vi "SPI_Read_protocol.vi"(0 "Register_adress":bool[](array[boolean])=[FALSE, FALSE, FALSE, FALSE, FALSE, FALSE, FALSE, FALSE, FALSE, FALSE, FALSE, FALSE, FALSE, FALSE, FALSE, FALSE, FALSE, FALSE, FALSE, FALSE, FALSE, FALSE, FALSE, FALSE, FALSE, FALSE, FALSE, FALSE, FALSE, FALSE, FALSE, FALSE], 1 "bit_index":i32, 3 "rising_edge":bool) -> (7 "SDO_Msg":bool)   [LabVIEW 2019]
doc: "This Vi Read a slave message based on SPI protocol. It works with a clock handler and inside a loop"
uses:
  <vilib>/rvi/eio/common/nirviEmuTemplateMethod_errors.vi
  <vilib>/eio/EIONode/EIONode.xnode
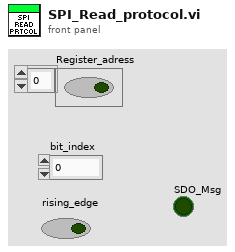
[diagram p1: front panel]
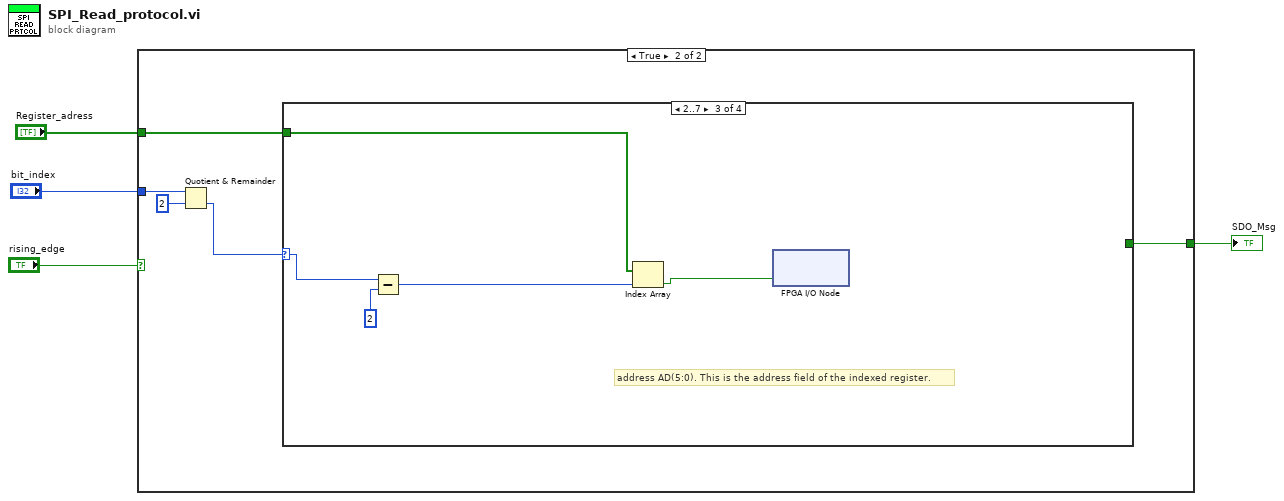
[diagram p0: block diagram]
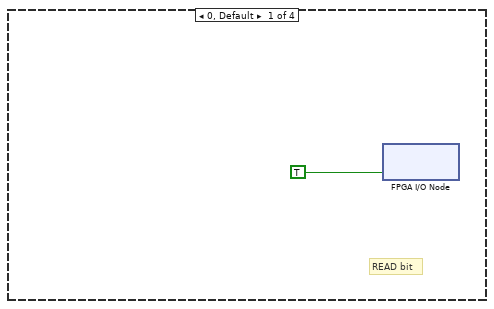
[diagram p3: hidden frame]
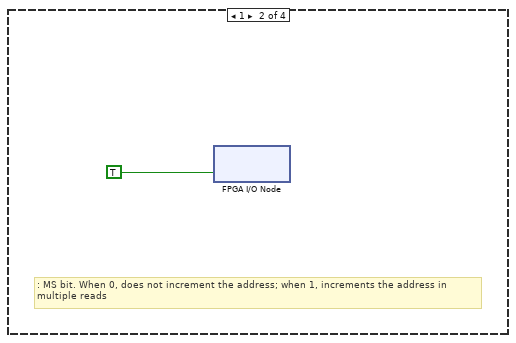
[diagram p4: hidden frame]
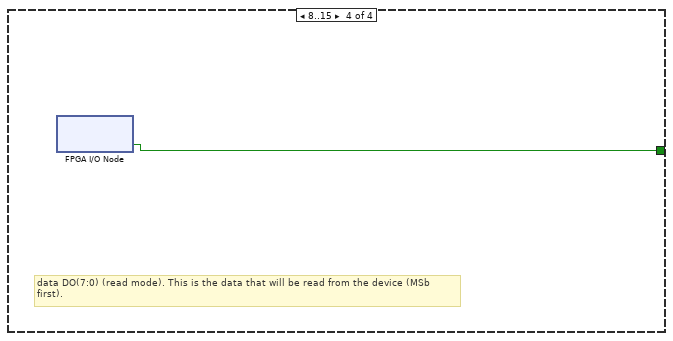
[diagram p5: hidden frame]
diagram:
  n1 = case shown="True" "rising_edge" {
    tunnel: "bit_index" -> [_ w8]
    tunnel: [_ w9] -> w2
    tunnel: "Register_adress" -> [_ w5]
    frame False {
    }
    frame True {
      n2 = Quotient & Remainder(x=w8, y=2) -> (floor(x/y)=w6:i32)  [unwired: 1 out]
      n3 = case shown="2..7" w6 {
        selector: w6 -> [_ _ w16 _]
        tunnel: [_ _ _ w17] -> w9
        tunnel: w5 -> [_ _ w13 _]
        frame 0, Default {
          # "READ bit"
          n4 = xnode "FPGA I/O Node"("SDI"=TRUE) -> ()  [unwired: 1 in, 1 out]
        }
        frame 1 {
          # ": MS bit. When 0, does not increment the address; when 1, increments the address in\nmultiple reads"
          n5 = xnode "FPGA I/O Node"("SDI"=TRUE) -> ()  [unwired: 1 in, 1 out]
        }
        frame 2..7 {
          # "address AD(5:0). This is the address field of the indexed register."
          n6 = Subtract(x=w16, y=2) -> (x-y=w14:i32)
          n7 = Index Array(array=w13, index=w14) -> (element=w12:bool)
          n8 = xnode "FPGA I/O Node"("SDI"=w12) -> ()  [unwired: 1 in, 1 out]
        }
        frame 8..15 {
          # "data DO(7:0) (read mode). This is the data that will be read from the device (MSb\nfirst)."
          n9 = xnode "FPGA I/O Node"() -> ("SDI"=w17:bool)  [unwired: 1 in, 1 out]
        }
      }
    }
  }
  "SDO_Msg" <- w2
